vi "InsertNewDeviceDB.vi"(8 "error in (no error)":errorcluster, 10 "DatabaseConnectionInfo":T1, 11 "Device name":string) -> (0 "error out":errorcluster)   [LabVIEW 2017]
uses:
  <vilib>/addons/database/Connection.llb/DB Tools Open Connec (Path).vi
  <vilib>/addons/database/NI_Database_API.lvlib
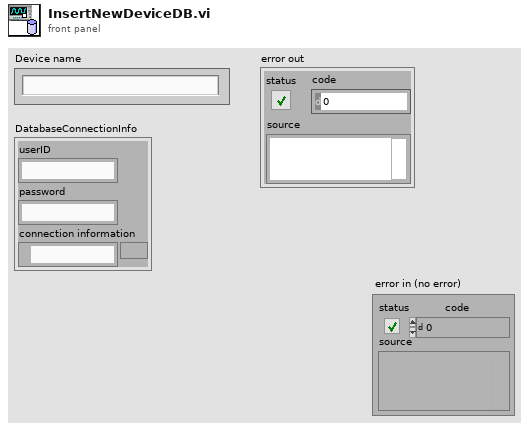
[diagram p1: front panel]
types:
  T1 = cluster{"userID":string, "password":string, "connection information":path}
  T2 = typedef "NI_Database_API.lvlib/Conn ObjectReference.ctl" = refnum<k1>
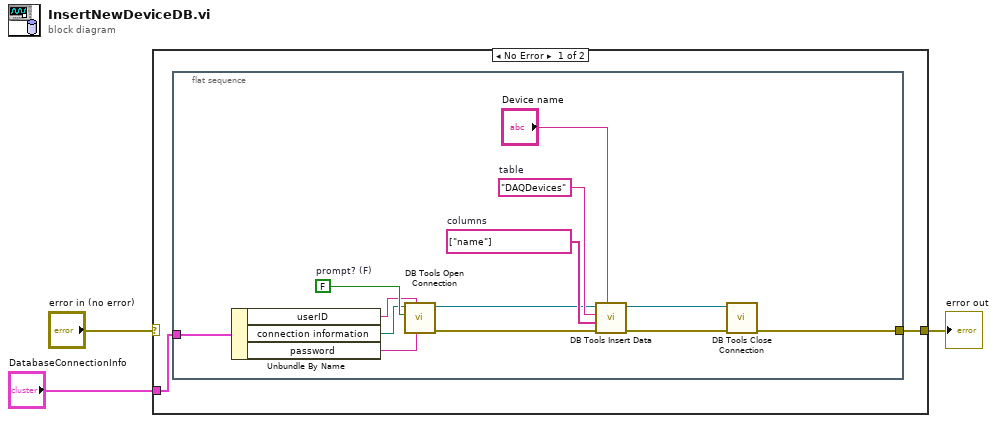
[diagram p0: block diagram]
diagram:
  n1 = case shown="No Error" "error in (no error)" {
    selector: "error in (no error)" -> [_ w19]
    tunnel: [w5 w19] -> w3
    tunnel: "DatabaseConnectionInfo" -> [w4 _]
    frame No Error {
      n2 = flat-sequence {
        tunnel: [w14] -> w5
        tunnel: w4 -> [w6]
        frame #0 {
          w12 = string[] ["name"]  # columns
          w13 = "DAQDevices"  # table
          w18 = FALSE  # prompt? (F)
          n3 = Unbundle By Name(w6) -> ("userID"=w17:string, "connection information"=w15:path, "password"=w16:string)
          n4 = call-poly <vilib>:"DB Tools Open Connection.vi"("password"=w16, "userID"=w17, "prompt? (F)"=w18, "connection information"=w15) -> ("error out"=w9:errorcluster, "connection reference"=w10:T2)  [unwired: 4 in]
          n5 = call <vilib>:"DB Tools Insert Data.vi"("data"="Device name", "error in (no error)"=w9, "columns"=w12, "table"=w13, "connection reference"=w10) -> ("error out"=w8:errorcluster, "connection reference out"=w7:T2)  [unwired: 5 in]
          n6 = call <vilib>:"DB Tools Close Connection.vi"("error in (no error)"=w8, "connection reference"=w7) -> ("error out"=w14:errorcluster)  [unwired: 5 in]
        }
      }
    }
    frame Error {
    }
  }
  "error out" <- w3
